vi "hse-application_SystemConfiguration.vi"(8 "error in":errorcluster, 11 "Application in":refnum<class "hse-application.lvclass">) -> (0 "error out":errorcluster, 3 "Application out":refnum<class "hse-application.lvclass">)   [LabVIEW 2014, in "hse-application.lvclass"]
doc: "Reads global (system-wide) configuration parameters from the config.ini file or creates it if it couldn't be found.\n\n\n\n____\nHAMPEL SOFTWARE ENGINEERING v0.12.0 (2018-09-13 18:21)"
uses:
  hse-application.lvclass
  hse-application.lvclass/hse-application.ctl
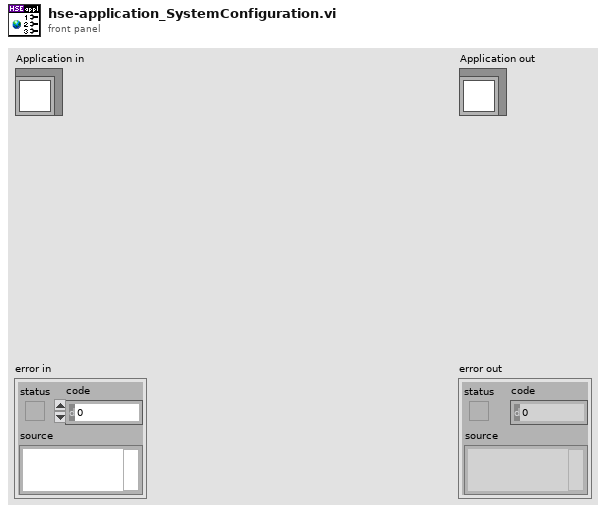
[diagram p1: front panel]
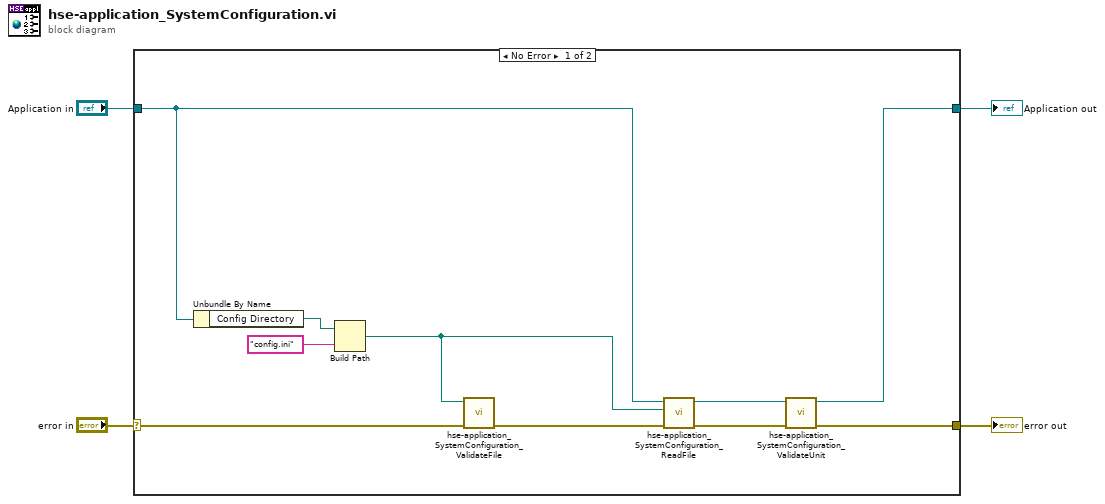
[diagram p0: block diagram]
diagram:
  n1 = case shown="No Error" "error in" {
    selector: "error in" -> [w13 w16]
    tunnel: [w7 w16] -> w3
    tunnel: [w5 w15] -> w1
    tunnel: "Application in" -> [w14 w15]
    frame No Error {
      n2 = Unbundle By Name(w14) -> ("Config Directory"=w10:path)
      n3 = Build Path(base path=w10, name or relative path="config.ini" ("Substring")) -> (appended path=w9:path)
      n4 = call "hse-application_SystemConfiguration_ValidateFile.vi"("error in (no error)"=w13, "Config File"=w9) -> ("error out"=w12:errorcluster)  [unwired: 9 in]
      n5 = call "hse-application_SystemConfiguration_ReadFile.vi"("error in (no error)"=w12, "Config File"=w9, "hse-application in"=w14) -> ("error out"=w8:errorcluster, "hse-application out"=w6:refnum<class "hse-application.lvclass">)  [unwired: 7 in]
      n6 = call "hse-application_SystemConfiguration_ValidateUnit.vi"("error in (no error)"=w8, "hse-application in"=w6) -> ("error out"=w7:errorcluster, "hse-application DUP"=w5:refnum<class "hse-application.lvclass">)  [unwired: 8 in]
    }
    frame Error {
    }
  }
  "error out" <- w3
  "Application out" <- w1
